vi "3D Coordinate Conversion (Array).vi"(8 "conversion type":u16(ring) items=["Cartesian to spherical", "spherical to Cartesian", "Cartesian to cylindrical", "cylindrical to Cartesian", "spherical to cylindrical", "cylindrical to spherical"], 9 "Axis 3":dbl[](array[numeric]), 10 "Axis 2":dbl[](array[numeric]), 11 "Axis 1":dbl[](array[numeric])) -> (0 "error":i32, 1 "Axis 3 Out":dbl[](array[numeric]), 2 "Axis 2 Out":dbl[](array[numeric]), 3 "Axis 1 Out":dbl[](array[numeric]))   [LabVIEW 2017, in "NI_AALPro.lvlib"]
doc: "Converts coordinates between the Cartesian, spherical, and cylindrical coordinate systems. Wire data to the <B>Axis 1</B> input to determine the polymorphic instance to use or manually select the instance."
uses:
  <vilib>/Analysis/NI_AALPro.lvlib
  <resource>/lvanlys.dll
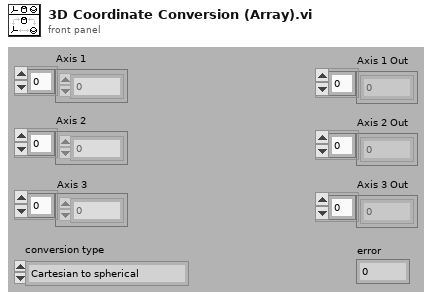
[diagram p1: front panel]
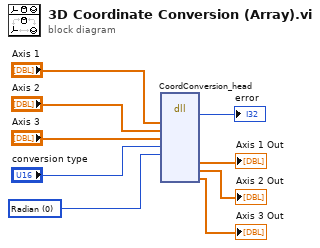
[diagram p0: block diagram]
diagram:
  w5 = u16 0 items=["Radian", "Degree"] ("unit")
  n1 = dll-call lib="e:/builds/penguin/labview/branches/2017/dev/dist/resource/lvanlys.*" fn="CoordConversion_head"("Axis1"="Axis 1", "Axis2"="Axis 2", "Axis3"="Axis 3", "ConversionType"="conversion type", "unit"=w5) -> (→"error":i32, "AxisOut1"=→"Axis 1 Out":dbl[], "AxisOut2"=→"Axis 2 Out":dbl[], "AxisOut3"=→"Axis 3 Out":dbl[])  [unwired: 11 in, 2 out]
